vi "Main.vi"(8 "error in":errorcluster, 11 "Opener in":refnum<class "Opener.lvclass">) -> (0 "error out":errorcluster, 3 "Opener out":refnum<class "Opener.lvclass">)   [LabVIEW 2020, in "Opener.lvclass"]
doc: "The Queued Message Handler of a Worker."
uses:
  Opener.lvclass
  <vilib>/addons/_Workers/Library/Classes/EHL/EHL.lvclass
  <vilib>/addons/_Workers/Library/Classes/Worker/Worker.lvclass
  <vilib>/addons/_Workers/Library/Classes/Error Handler/Error Handler.lvclass
  Initialization Data.ctl
  C:/Program Files (x86)/National Instruments/LabVIEW 2020/vi.lib/addons/_Workers/Library/Classes/Worker/Worker.lvclass
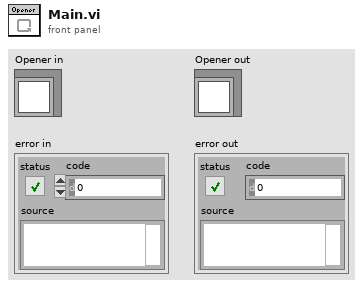
[diagram p1: front panel]
types:
  T1 = typedef "Opener.lvclass/Initialization Data.ctl" = cluster{"String":string}
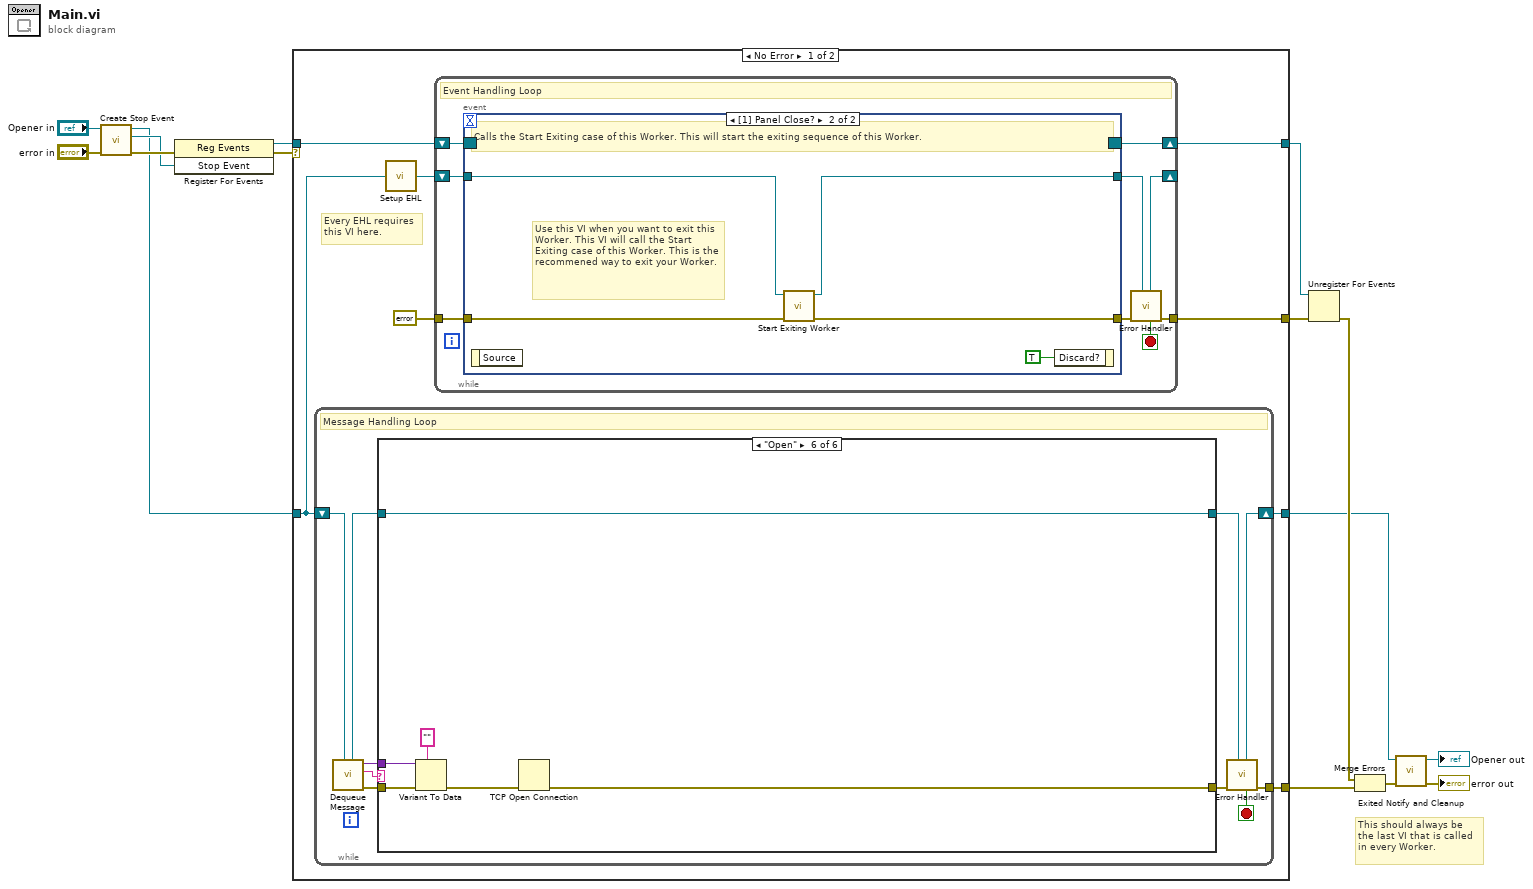
[diagram p0: block diagram]
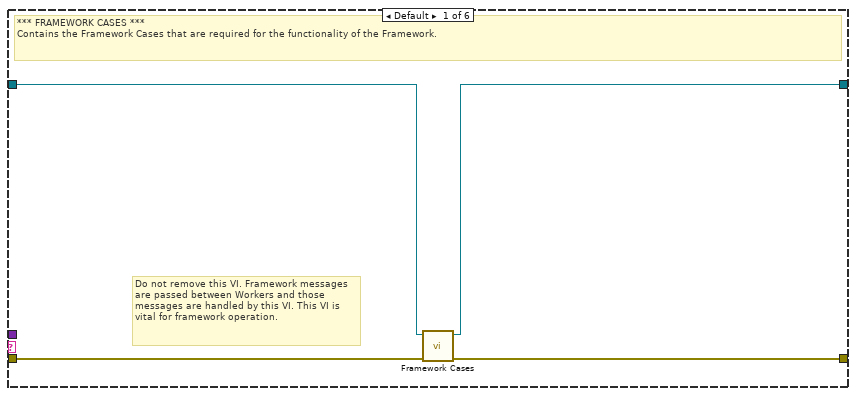
[diagram p2: hidden frame]
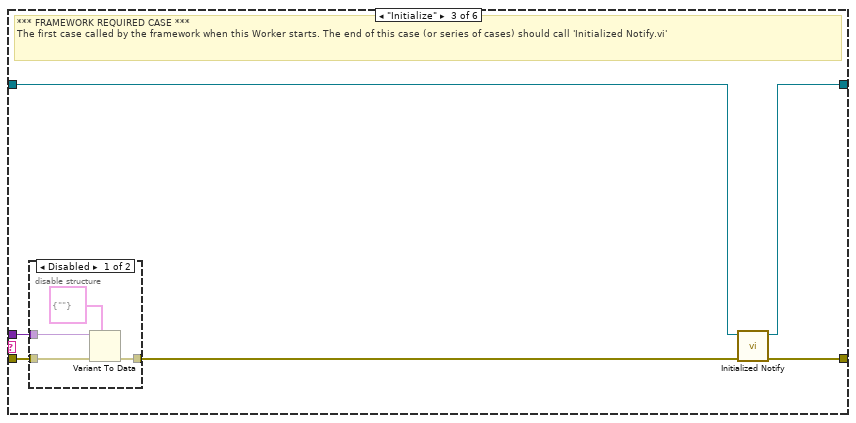
[diagram p4: hidden frame]
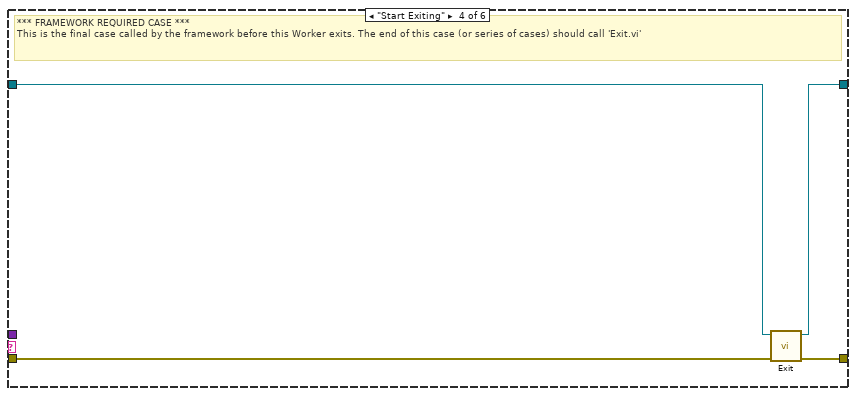
[diagram p6: hidden frame]
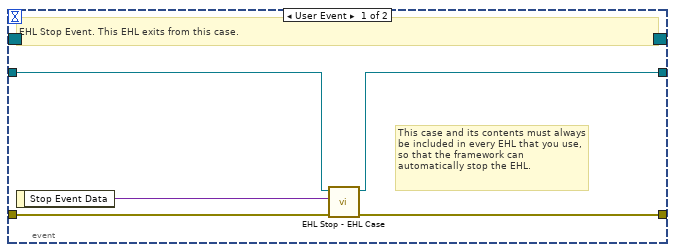
[diagram p8: hidden frame]
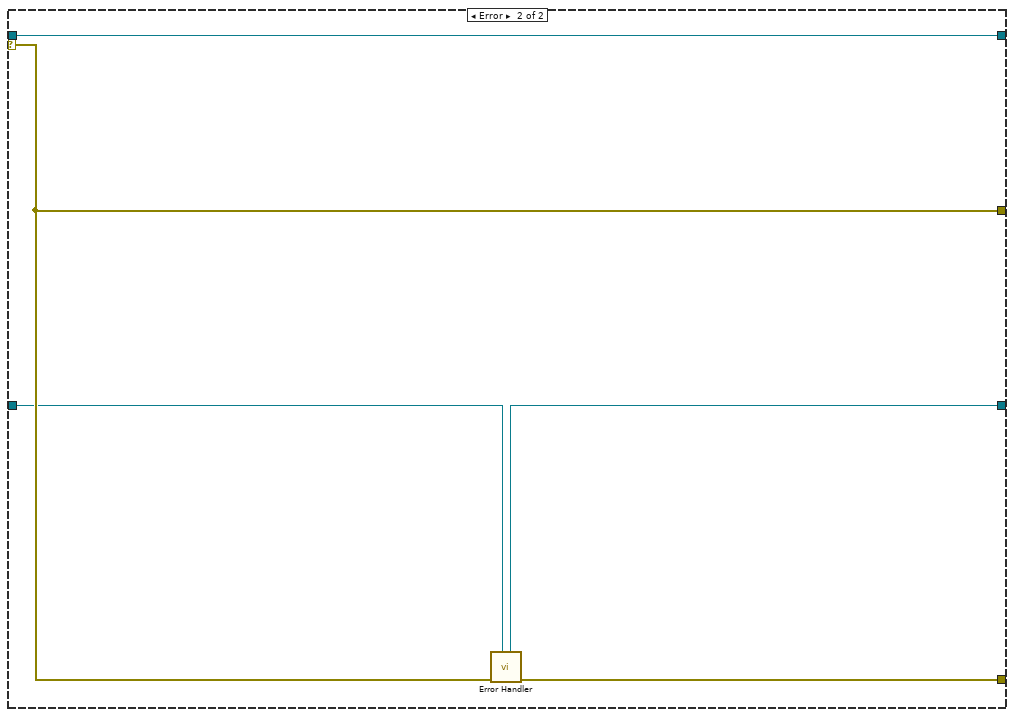
[diagram p9: hidden frame]
diagram:
  # "This should always be the last VI that is called in every Worker."
  n1 = call <vilib>:"Create Stop Event.vi"("error in"="error in", "Worker"="Opener in") -> ("error out"=w10:errorcluster, "Stop Event"=w7:refnum<user-event>, "Worker out"=w4:refnum<class "Opener.lvclass">)  [unwired: 7 in]
  n2 = register-events(error in=w10, w7) -> (reference out=w9:refnum<event-registration>, error out=w1:errorcluster)  [unwired: 1 in]
  n3 = case shown="No Error" w1 {
    tunnel: w4 -> [w18 w83]
    tunnel: [w16 w84] -> w8
    tunnel: w9 -> [w23 w85]
    tunnel: [w20 w86] -> w14
    tunnel: [w22 w85] -> w13
    tunnel: [w17 w82] -> w11
    selector: w1 -> [_ w86]
    frame No Error {
      # "Every EHL requires\nthis VI here."
      n4 = while {
        shift-right: [w31] -> w17
        shift-left: w18 -> [w33]
        tunnel: [w32] -> w16
        stop <- w24 stop-if-true
        # "Message Handling Loop"
        n5 = call <vilib>:"Dequeue Message.vi"("Worker"=w33) -> ("error out"=w30:errorcluster, "Case out"=w25:string, "Data out"=w26:variant, "Worker out"=w28:refnum<class "Opener.lvclass">)  [unwired: 6 in, 1 out]
        n6 = case "WORKERS MHL Case Structure (DO NOT CHANGE LABEL NAME)" shown="\"Open\"" w25 {
          tunnel: w30 -> [w37 w38 w43 w51 w55 w62]
          tunnel: [w36 w38 w45 w54 w55 w58] -> w29
          tunnel: w28 -> [w35 w39 w42 w52 w56 w61]
          tunnel: [w34 w39 w44 w53 w56 w61] -> w27
          tunnel: w26 -> [_ _ w40 _ _ w59]
          frame Default {
            # "Do not remove this VI. Framework messages are passed between Workers and those messages are handled by this VI. This VI is vital for framework operation."
            # "*** FRAMEWORK CASES ***\nContains the Framework Cases that are required for the functionality of the Framework."
            n7 = call <vilib>:"Framework Cases.vi"("error in"=w37, "Worker"=w35) -> ("error out"=w36:errorcluster, "Worker out"=w34:refnum<class "Opener.lvclass">)  [unwired: 8 in]
          }
          frame "------ FRAMEWORK REQUIRED CASES ------" {
            # "Start of Framework Required Cases"
          }
          frame "Initialize" {
            # "*** FRAMEWORK REQUIRED CASE ***\nThe first case called by the framework when this Worker starts. The end of this case (or series of cases) should call 'Initialized Notify.vi'"
            n8 = disable-structure shown="Disabled" {
              disable-tunnel: w43 -> [w49 w50]
              disable-tunnel: [w48 w50] -> w41
              disable-tunnel: w40 -> [w47 _]
              frame Disabled {
                n9 = Variant To Data(error in=w49, type=T1 {"String"=""} ("Initialization Data"), Variant=w47) -> (error out=w48:errorcluster)  [unwired: 1 out]
              }
              frame Enabled {
              }
            }
            n10 = call <vilib>:"Initialized Notify.vi"("error in"=w41, "Worker"=w42) -> ("error out"=w45:errorcluster, "dup Worker out"=w44:refnum<class "Opener.lvclass">)  [unwired: 8 in]
          }
          frame "Start Exiting" {
            # "*** FRAMEWORK REQUIRED CASE ***\nThis is the final case called by the framework before this Worker exits. The end of this case (or series of cases) should call 'Exit.vi'"
            n11 = call <vilib>:"Exit.vi"("error_in"=w51, "Worker"=w52) -> ("error out"=w54:errorcluster, "dup Worker out"=w53:refnum<class "Opener.lvclass">)  [unwired: 8 in]
          }
          frame "-----------------------------------------------" {
            # "End of Framework Required Cases"
          }
          frame "Open" {
            n12 = Variant To Data(error in=w62, type="", Variant=w59) -> (error out=w60:errorcluster)  [unwired: 1 out]
            n13 = TCP Open Connection(error in (no error)=w60) -> (error out=w58:errorcluster)  [unwired: 4 in, 1 out]
          }
        }
        n14 = call <vilib>:"Error Handler.vi"("Worker"=w27, "error_in"=w29) -> ("error out"=w32:errorcluster, "Stop Loop"=w24:bool, "Worker out"=w31:refnum<class "Opener.lvclass">)  [unwired: 7 in]
      }
      n15 = call <vilib>:"Setup EHL.vi"("Worker"=w18) -> ("Worker out"=w19:refnum<class "Opener.lvclass">)  [unwired: 14 in]
      n16 = while "Event Handling Loop" {
        shift-right: [w71] -> w22
        shift-left: w23 -> [w70]
        tunnel: [w66] -> w20
        tunnel: errorcluster {"status"=FALSE, "code"=0, "source"=""} ("error constant") -> [w68]
        shift-right: [w64] -> _
        shift-left: w19 -> [w69]
        stop <- w63 stop-if-true
        # "Event Handling Loop"
        n17 = event shown="[1] Panel Close?" {
          selector: w70 -> [_ _]
          dyn-events: [_ _] -> w71
          timeout: _ -> [_ _]
          tunnel: [w75 w80] -> w67
          tunnel: w68 -> [w76 w79]
          tunnel: w69 -> [w74 w78]
          tunnel: [w73 w77] -> w65
          event User Event {
            # "This case and its contents must always be included in every EHL that you use, so that the framework can automatically stop the EHL."
            # "EHL Stop Event. This EHL exits from this case."
            n18 = event-data() -> ("Stop Event Data"=w72:variant)  [unwired: 1 in]
            n19 = call <vilib>:"EHL Stop - EHL Case.vi"("error in"=w76, "Stop Event Data"=w72, "Worker"=w74) -> ("error out"=w75:errorcluster, "Worker out"=w73:refnum<class "Opener.lvclass">)  [unwired: 7 in]
          }
          event Panel Close? {
            # "Use this VI when you want to exit this Worker. This VI will call the Start Exiting case of this Worker. This is the recommened way to exit your Worker."
            # "Calls the Start Exiting case of this Worker. This will start the exiting sequence of this Worker."
            n20 = event-data() -> ()  [unwired: 1 in, 1 out]
            n21 = call <vilib>:"Start Exiting Worker.vi"("error in"=w79, "Worker"=w78) -> ("error out"=w80:errorcluster, "dup Worker out"=w77:refnum<class "Opener.lvclass">)  [unwired: 8 in]
            n22 = event-data("Discard?"=TRUE) -> ()  [unwired: 1 in, 1 out]
          }
        }
        n23 = call <vilib>:"Error Handler.vi"("Worker"=w65, "error_in"=w67) -> ("error out"=w66:errorcluster, "Stop Loop"=w63:bool, "Worker out"=w64:refnum<class "Opener.lvclass">)  [unwired: 7 in]
      }
    }
    frame Error {
      n24 = call <vilib>:"Error Handler.vi"("Worker"=w83, "error_in"=w86) -> ("error out"=w84:errorcluster, "Worker out"=w82:refnum<class "Opener.lvclass">)  [unwired: 7 in, 1 out]
    }
  }
  n25 = Unregister For Events(event registration refnum=w13, error in=w14) -> (error out=w15:errorcluster)
  n26 = Merge Errors(w15, w8) -> (w12:errorcluster)
  n27 = call <vilib>:"Exited Notify and Cleanup.vi"("error_in"=w12, "Worker"=w11) -> ("error out"=→"error out":errorcluster, "dup Worker out"=→"Opener out":refnum<class "Opener.lvclass">)  [unwired: 8 in]
